vi "Main Process Case.vi"(8 "error in (no error)":errorcluster, 10 "CurrentAction":string, 11 "Main Process Class in":refnum<class "Main Class.lvclass">) -> (0 "error out":errorcluster, 1 "KeepCase":bool, 3 "Main Process Class out":refnum<class "Main Class.lvclass">)   [LabVIEW 2019, in "Main Class.lvclass"]
uses:
  Main Class.lvclass
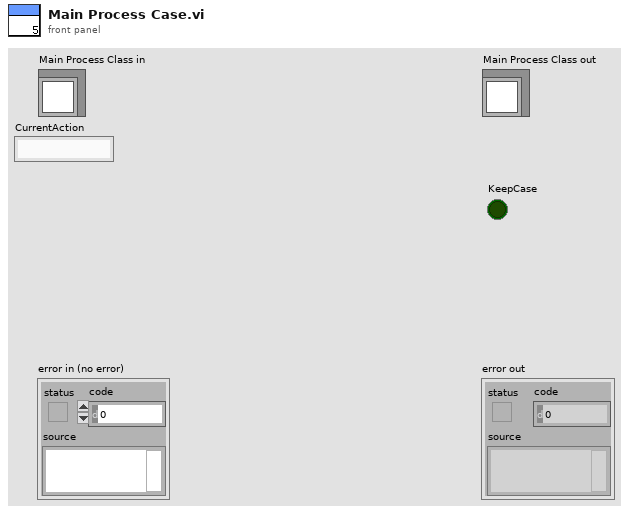
[diagram p1: front panel]
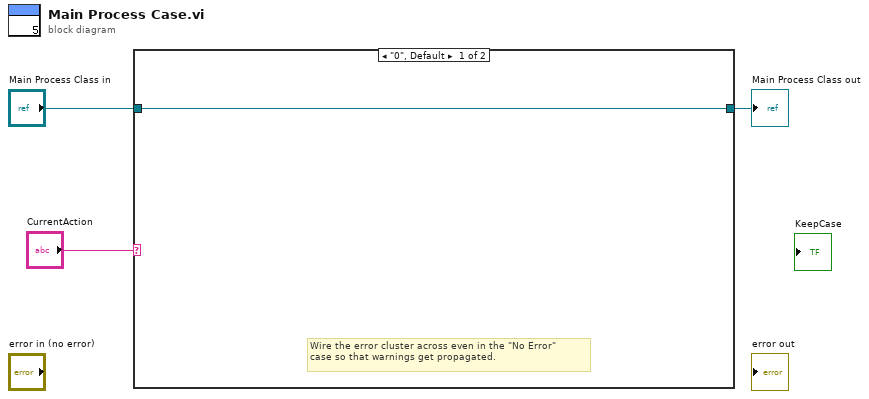
[diagram p0: block diagram]
diagram:
  n1 = case shown="\"0\", Default" "CurrentAction" {
    tunnel: [w4 w5] -> w2
    tunnel: "Main Process Class in" -> [w4 w5]
    frame "0", Default {
      # "Wire the error cluster across even in the \"No Error\"\ncase so that warnings get propagated."
    }
    frame "1" {
    }
  }
  "Main Process Class out" <- w2
